vi "New Experiment Dialog.vi"(8 "error in (no error)":errorcluster, 10 "Experiment Location":path, 11 "Experiment Name":string) -> (0 "error out":errorcluster, 1 "cancelled":bool, 2 "Project Directory out":path, 3 "Project Name out":string)   [LabVIEW 2020, in "Experiment Manager.lvlib"]
doc: "Opens a dialog window to specify the name and folder location of a new experiment. Project Name and Project Location will be blank if values are not provided, and any values provided will be validated and the dialog updated accordingly."
uses:
  Experiment Manager.lvlib
  New Experiment Dialog Data.ctl
panel:
  out "Experiment Directory Status":string="Invalid path provided."
  out "Experiment Name Status":string
  in  "Cancel Btn":bool
  in  "OK Btn":bool
  # "Create New Experiment"
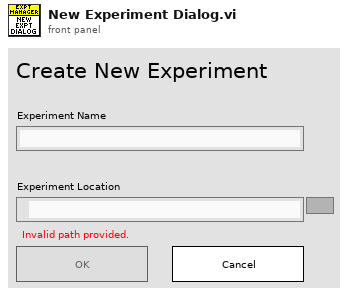
[diagram p1: front panel]
types:
  T1 = enum8{"Enabled", "Disabled", "Disabled and Grayed Out"}
  T2 = typedef "Experiment Manager.lvlib/New Experiment Dialog Data.ctl" = cluster{"Is name valid?":bool, "Is directory valid?":bool}
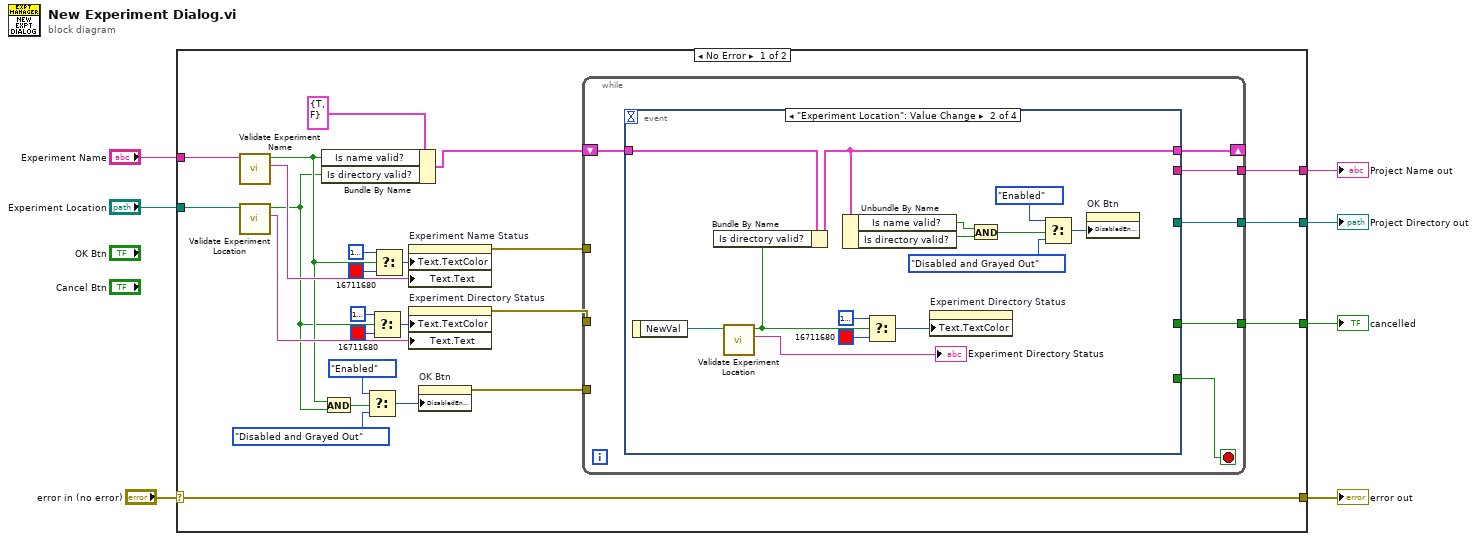
[diagram p0: block diagram]
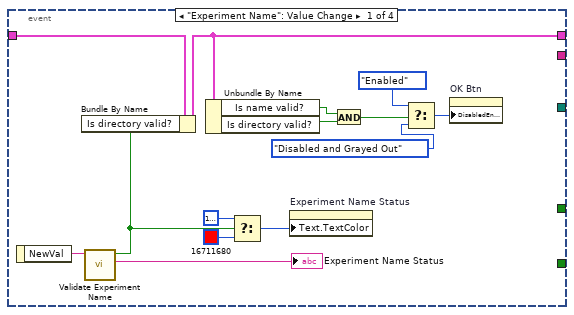
[diagram p2: hidden frame]
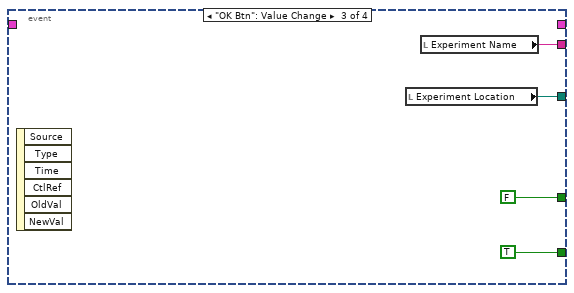
[diagram p3: hidden frame]
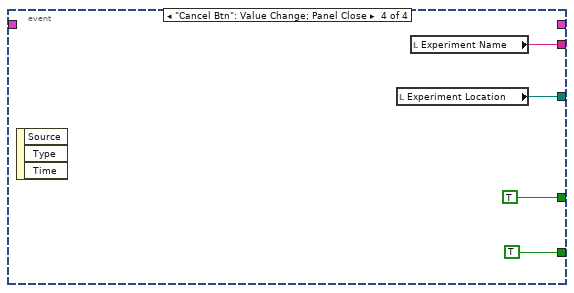
[diagram p4: hidden frame]
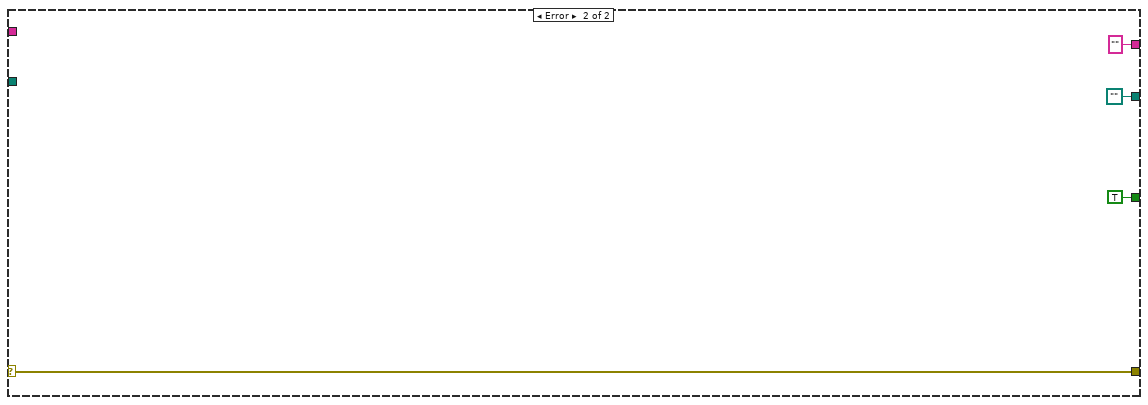
[diagram p5: hidden frame]
diagram:
  n1 = case shown="No Error" "error in (no error)" {
    selector: "error in (no error)" -> [w29 w78]
    tunnel: [w29 w78] -> w6
    tunnel: [w28 path ""] -> w5
    tunnel: [w27 "" ("Project Name")] -> w4
    tunnel: "Experiment Name" -> [w26 _]
    tunnel: "Experiment Location" -> [w25 _]
    tunnel: [w8 TRUE] -> w1
    frame No Error {
      n2 = call "Validate Experiment Name.vi"("Experiment Name"=w26) -> ("Error (if invalid)"=w23:string, "Valid Experiment Name?"=w10:bool)  [unwired: 9 in]
      n3 = call "Validate Experiment Location.vi"("Experiment Location"=w25) -> ("Error (if invalid)"=w22:string, "Valid Experiment Directory?"=w9:bool)  [unwired: 9 in]
      n4 = Bundle By Name(cluster=T2 {"Is name valid?"=TRUE, "Is directory valid?"=FALSE}, "Is name valid?"=w10, "Is directory valid?"=w9) -> (w15:T2)
      n5 = And(x=w10, y=w9) -> (x .and. y?=w14:bool)
      n6 = Select(t=T1."Enabled" ("Disabled"), s=w14, f=T1."Disabled and Grayed Out" ("Disabled")) -> (s? t:f=w11:T1)
      n7 = Select(t=u32 16777228, s=w9, f=u32 16711680) -> (s? t:f=w16:u32)
      n8 = Select(t=u32 16777228, s=w10, f=u32 16711680) -> (s? t:f=w19:u32)
      n9 = property on="Experiment Name Status" class="Str"("Text.TextColor"=w19, "Text.Text"=w23) -> (error out=w32:errorcluster)  [unwired: 2 in, 1 out]
      n10 = property on="Experiment Directory Status" class="Str"("Text.TextColor"=w16, "Text.Text"=w22) -> (error out=w31:errorcluster)  [unwired: 2 in, 1 out]
      n11 = property on="OK Btn" class="Bool"("DisabledEnum"=w11) -> (error out=w30:errorcluster)  [unwired: 2 in, 1 out]
      n12 = while {
        tunnel: [w38] -> w27
        tunnel: [w37] -> w28
        shift-right: [w34] -> _
        shift-left: w15 -> [w35]
        tunnel: w32 -> [_]
        tunnel: w31 -> [_]
        tunnel: w30 -> [_]
        tunnel: [w33] -> w8
        stop <- w36 stop-if-true
        n13 = event shown="[1] \"Experiment Location\": Value Change" {
          selector: _ -> [_ _ _ _]
          dyn-events: _ -> [_ _ _ _]
          timeout: _ -> [_ _ _ _]
          tunnel: [_ _ w68 w72] -> w38
          tunnel: [_ _ w69 w71] -> w37
          tunnel: [_ _ TRUE TRUE] -> w36
          tunnel: [w40 w60 _ _] -> w34
          tunnel: w35 -> [w42 w62 _ _]
          tunnel: [_ _ FALSE TRUE] -> w33
          event "Experiment Name": Value Change {
            n14 = event-data() -> ("NewVal"=w39:string)  [unwired: 1 in]
            n15 = call "Validate Experiment Name.vi"("Experiment Name"=w39) -> ("Error (if invalid)"=→"Experiment Name Status":string, "Valid Experiment Name?"=w41:bool)  [unwired: 9 in]
            n16 = Bundle By Name(cluster=w42, "Is directory valid?"=w41) -> (w40:T2)
            n17 = Unbundle By Name(w40) -> ("Is name valid?"=w48:bool, "Is directory valid?"=w47:bool)
            n18 = Select(t=u32 16777228, s=w41, f=u32 16711680) -> (s? t:f=w50:u32)
            n19 = property on="Experiment Name Status" class="Str"("Text.TextColor"=w50) -> ()  [unwired: 2 in, 2 out]
            n20 = And(x=w48, y=w47) -> (x .and. y?=w46:bool)
            n21 = Select(t=T1."Enabled" ("Disabled"), s=w46, f=T1."Disabled and Grayed Out" ("Disabled")) -> (s? t:f=w45:T1)
            n22 = property on="OK Btn" class="Bool"("DisabledEnum"=w45) -> ()  [unwired: 2 in, 2 out]
          }
          event "Experiment Location": Value Change {
            n23 = event-data() -> ("NewVal"=w53:path)  [unwired: 1 in]
            n24 = call "Validate Experiment Location.vi"("Experiment Location"=w53) -> ("Error (if invalid)"=→"Experiment Directory Status":string, "Valid Experiment Directory?"=w61:bool)  [unwired: 9 in]
            n25 = Bundle By Name(cluster=w62, "Is directory valid?"=w61) -> (w60:T2)
            n26 = Unbundle By Name(w60) -> ("Is name valid?"=w59:bool, "Is directory valid?"=w58:bool)
            n27 = Select(t=u32 16777228, s=w61, f=u32 16711680) -> (s? t:f=w63:u32)
            n28 = property on="Experiment Directory Status" class="Str"("Text.TextColor"=w63) -> ()  [unwired: 2 in, 2 out]
            n29 = And(x=w59, y=w58) -> (x .and. y?=w57:bool)
            n30 = Select(t=T1."Enabled" ("Disabled"), s=w57, f=T1."Disabled and Grayed Out" ("Disabled")) -> (s? t:f=w54:T1)
            n31 = property on="OK Btn" class="Bool"("DisabledEnum"=w54) -> ()  [unwired: 2 in, 2 out]
          }
          event "OK Btn": Value Change {
            n32 = event-data() -> ()  [unwired: 1 in, 6 out]
            n33 = local read "Experiment Location"() -> (w69:path)
            n34 = local read "Experiment Name"() -> (w68:string)
          }
          event "Cancel Btn": Value Change; Panel Close {
            n35 = event-data() -> ()  [unwired: 1 in, 3 out]
            n36 = local read "Experiment Location"() -> (w71:path)
            n37 = local read "Experiment Name"() -> (w72:string)
          }
        }
      }
    }
    frame Error {
    }
  }
  "error out" <- w6
  "Project Name out" <- w4
  "Project Directory out" <- w5
  "cancelled" <- w1
